vi "BLM_SetToValue.vi"(1 "Position":dbl min=-2147483647.0 max=2147483647.0 format="%#_10g", 2 "error in (no error)":errorcluster, 3 "Motor Address":string="0", 4 "Port Address":refnum<visa-resource-name>) -> (0 "error out":errorcluster)   [LabVIEW 2019]
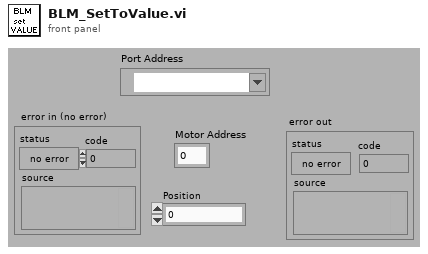
[diagram p1: front panel]
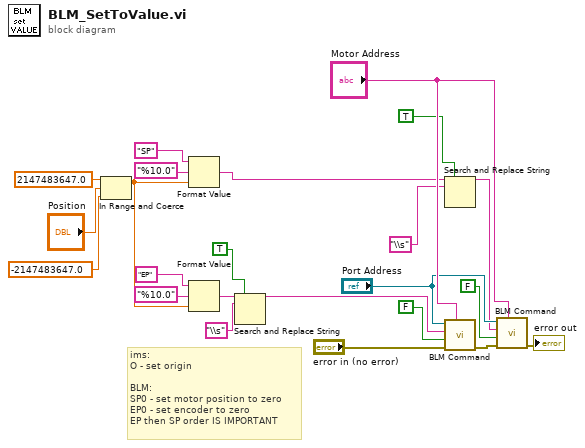
[diagram p0: block diagram]
diagram:
  # "ims:\nO - set origin\n\nBLM:\nSP0 - set motor position to zero\nEP0 - set encoder to zero\nEP then SP order IS IMPORTANT"
  n1 = In Range and Coerce(upper limit=2147483647.0 ("x"), x="Position", lower limit=-2147483647.0) -> (coerced(x)=w16:dbl)  [unwired: 1 out]
  n2 = Format Value(string ("")="SP", format string="%10.0", value (0)=w16) -> (output string=w8:string)
  n3 = Format Value(string ("")="EP", format string="%10.0", value (0)=w16) -> (output string=w5:string)
  n4 = Search and Replace String(replace all?=TRUE ("replace all? (F)"), input string=w5, search string="\\s") -> (result string=w4:string)  [unwired: 5 in, 3 out]
  n5 = Search and Replace String(replace all?=TRUE ("replace all? (F)"), input string=w8, search string="\\s") -> (result string=w9:string)  [unwired: 5 in, 3 out]
  n6 = call "BLM Command.vi"("Motor Address"="Motor Address", "error in (no error)"="error in (no error)", "Read Echo?"=FALSE, "Command"=w4, "Port Address"="Port Address") -> ("error out"=w14:errorcluster)  [unwired: 1 in, 4 out]
  n7 = call "BLM Command.vi"("Motor Address"="Motor Address", "error in (no error)"=w14, "Read Echo?"=FALSE, "Command"=w9, "Port Address"="Port Address") -> ("error out"=→"error out":errorcluster)  [unwired: 1 in, 4 out]
